vi "scale_manage.vi"(8 "error in (no error)":errorcluster, 11 "Graph_ref_in":refnum<vi>) -> (0 "error out":errorcluster, 3 "Graph_ref_out":refnum<vi>)   [LabVIEW 2020, in "GraphBG_manage.lvlib" / "Graph.lvclass"]
uses:
  Graph.lvclass
  T50/subVI/xyY_graph.ctl
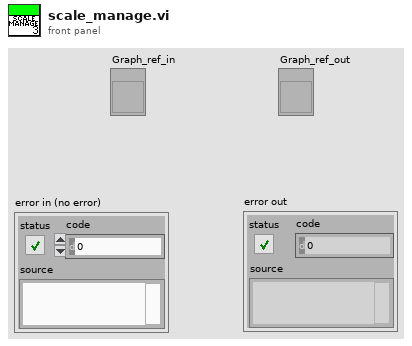
[diagram p1: front panel]
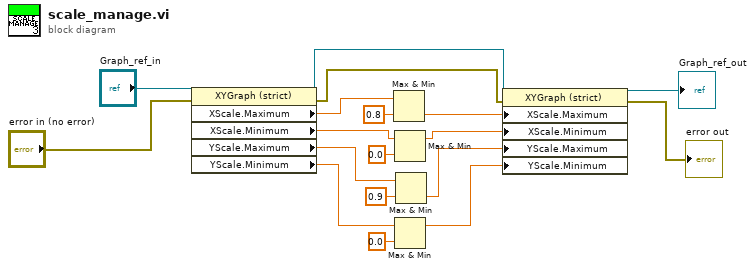
[diagram p0: block diagram]
diagram:
  n1 = property on="Property Node" class="XYGraph (strict)"(reference="Graph_ref_in", error in="error in (no error)") -> (reference out=w4:refnum<vi>, error out=w2:errorcluster, "XScale.Maximum"=w18:dbl, "XScale.Minimum"=w14:dbl, "YScale.Maximum"=w12:dbl, "YScale.Minimum"=w9:dbl)
  n2 = Max & Min(x=w18, y=0.8) -> (min(x,y)=w16:dbl)  [unwired: 1 out]
  n3 = Max & Min(x=w14, y=0.0) -> (max(x,y)=w13:dbl)  [unwired: 1 out]
  n4 = Max & Min(x=w9, y=0.0) -> (max(x,y)=w7:dbl)  [unwired: 1 out]
  n5 = Max & Min(x=w12, y=0.9) -> (min(x,y)=w11:dbl)  [unwired: 1 out]
  n6 = property on="Property Node" class="XYGraph (strict)"(reference=w4, error in=w2, "XScale.Maximum"=w16, "XScale.Minimum"=w13, "YScale.Maximum"=w11, "YScale.Minimum"=w7) -> (reference out=→"Graph_ref_out":refnum<vi>, error out=→"error out":errorcluster)
